vi "Example 3.vi"   [LabVIEW 2018]
uses:
  <vilib>/addons/VeriStand Custom Device Scripting APIs/FPGA Addon/Scripting API.lvlib
  <vilib>/addons/VeriStand Custom Device Scripting APIs/FPGA Addon/TypeDefs/Input Scalar Data.ctl
  <vilib>/addons/VeriStand Custom Device Scripting APIs/FPGA Addon/Private/Import Bitfile Scalars (Instances)/Import Scalars - by label.vi
types:
  T1 = typedef "Scripting API.lvlib/Input Scalar Data.ctl" = cluster{"Bitfile Name":string, "SysDef Name":string}
  T2 = typedef "Custom Device API.lvlib/Custom Device Item Ref.ctl" = u64
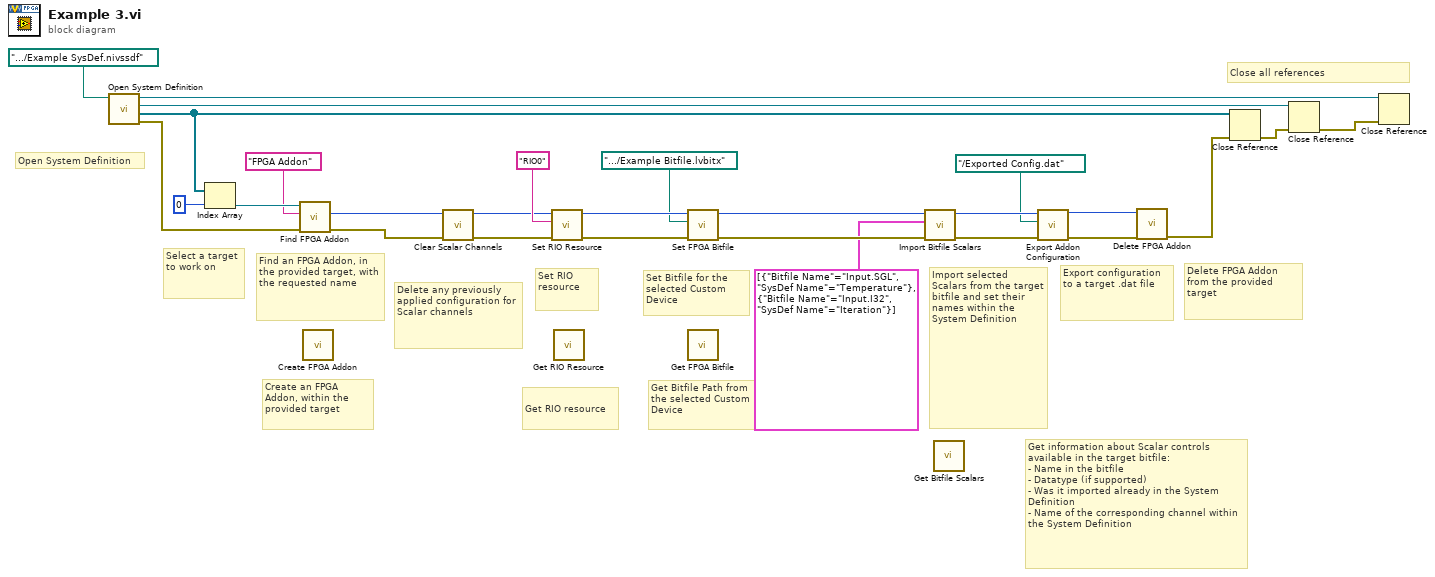
[diagram p0: block diagram]
diagram:
  # "Delete any previously applied configuration for Scalar channels"
  # "Delete FPGA Addon from the provided target"
  # "Export configuration to a target .dat file"
  # "Create an FPGA Addon, within the provided target"
  # "Get information about Scalar controls  available in the target bitfile:\n- Name in the bitfile\n- Datatype (if supported)\n- Was it imported already in the System Definition\n- Name of the corresponding channel within the System Definition"
  # "Get Bitfile Path from the selected Custom Device"
  # "Get RIO resource"
  # "Import selected Scalars from the target bitfile and set their names within the System Definition"
  # "Close all references"
  # "Set Bitfile for the selected Custom Device"
  # "Set RIO resource"
  # "Find an FPGA Addon, in the provided target, with the requested name"
  # "Select a target to work on"
  # "Open System Definition"
  n1 = call <vilib>:"Open System Definition.vi"("System Definition File"=path ".../Example SysDef.nivssdf" ("fpga bitfile path")) -> ("error out"=w13:errorcluster, "targets refnums"=w17:refnum<k24>[], "root refnum"=w18:refnum<k24>, "system definition refnum"=w19:refnum<k24>)  [unwired: 7 in]
  n2 = Index Array(array=w17, index=0) -> (element=w12:refnum<k24>)
  n3 = call <vilib>:"Find FPGA Addon.vi"("error in (no error)"=w13, "fpga addon name"="FPGA Addon", "target in"=w12) -> ("error out"=w3:errorcluster, "fpga addon refnum out"=w4:T2)  [unwired: 5 in, 2 out]
  n4 = call <vilib>:"Create FPGA Addon.vi"() -> ()  [unwired: 9 in, 3 out]
  n5 = call <vilib>:"Clear Scalar Channels.vi"("error in (no error)"=w3, "fpga addon refnum in"=w4) -> ("error out"=w2:errorcluster, "fpga addon refnum out"=w1:T2)  [unwired: 8 in]
  n6 = call <vilib>:"Set RIO Resource.vi"("error in (no error)"=w2, "rio resource in"="RIO0", "fpga addon refnum in"=w1) -> ("error out"=w25:errorcluster, "fpga addon refnum out"=w24:T2)  [unwired: 7 in]
  n7 = call <vilib>:"Get RIO Resource.vi"() -> ()  [unwired: 9 in, 3 out]
  n8 = call <vilib>:"Set FPGA Bitfile.vi"("error in (no error)"=w25, "fpga bitfile path"=path ".../Example Bitfile.lvbitx", "fpga addon refnum in"=w24) -> ("error out"=w21:errorcluster, "fpga addon refnum out"=w20:T2)  [unwired: 7 in]
  n9 = call <vilib>:"Get FPGA Bitfile.vi"() -> ()  [unwired: 9 in, 3 out]
  n10 = call-poly <vilib>:"Import Bitfile Scalars.vi"("error in (no error)"=w21, "bitfile scalars in"=T1[] [{"Bitfile Name"="Input.SGL", "SysDef Name"="Temperature"}, {"Bitfile Name"="Input.I32", "SysDef Name"="Iteration"}], "fpga addon refnum in"=w20) -> ("error out"=w10:errorcluster, "fpga addon refnum out"=w9:T2)  [unwired: 6 in, 1 out]
  n11 = call <vilib>:"Get Bitfile Scalars.vi"() -> ()  [unwired: 9 in, 3 out]
  n12 = call <vilib>:"Export Addon Configuration.vi"("error in (no error)"=w10, "export file path"=path "../Exported Config.dat", "fpga addon refnum in"=w9) -> ("error out"=w7:errorcluster, "fpga addon refnum out"=w6:T2)  [unwired: 7 in]
  n13 = call <vilib>:"Delete FPGA Addon.vi"("error in (no error)"=w7, "fpga addon refnum"=w6) -> ("error out"=w5:errorcluster)  [unwired: 9 in]
  n14 = Close Reference(reference=w17, error in (no error)=w5) -> (error out=w16:errorcluster)
  n15 = Close Reference(reference=w18, error in (no error)=w16) -> (error out=w15:errorcluster)
  n16 = Close Reference(reference=w19, error in (no error)=w15) -> ()  [unwired: 1 out]
